vi "ClientGUIMonitorAllAnalog.vi"() -> ()   [LabVIEW 2021]
doc: "Le protocole UDP diffère du protocole TCP car il n'y a pas de détection d'erreur avec les paquets d'informations qui sont envoyés ; il n'y a donc aucune garantie qu'un destinataire reçoive bien des données.\n\nLe protocole UDP offre la possibilité de diffuser des données sur un réseau. Spécifiez simplement une adresse IP de uns (255.255.255.255) pour essayer de diffuser l'information sur tout le réseau. Gardez à l'esprit que des routeurs et d'autres périphériques de réseau refusent généralement de diffuser au-delà de certains points, la diffusion est donc limitée dans la pratique."
panel:
  out "Value":u16
  in  "?":bool
  in  "Période\n(en ds)":u32(slide)=100 min=5 max=100 step=5 scale=5.0..100.0
  out "Pin0":u16(graph)
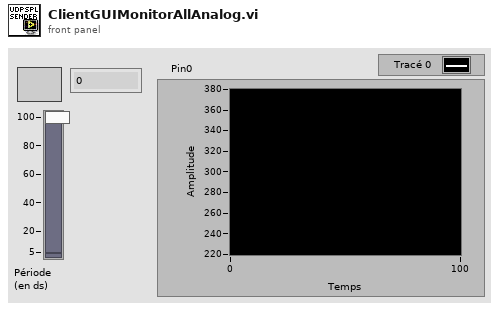
[diagram p1: front panel]
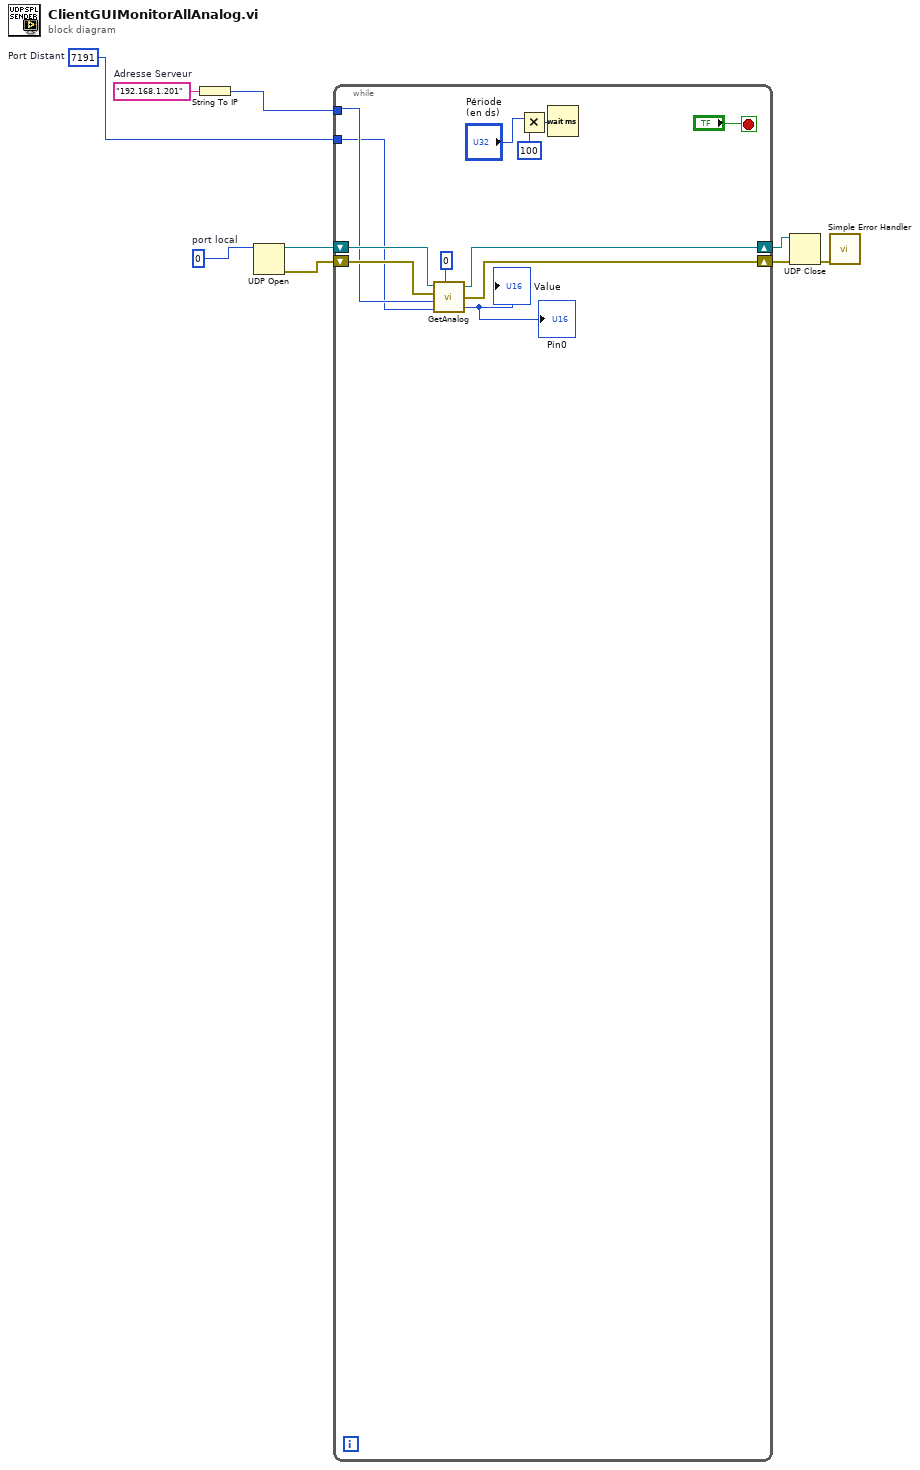
[diagram p0: block diagram]
diagram:
  w7 = u16 7191  # Port Distant
  w6 = "192.168.1.201"  # Adresse Serveur
  w9 = u16 0  # port local
  n1 = String To IP(1:w6) -> (0:w8:u32)
  n2 = UDP Open(11:w9) -> (port=w5:refnum<k16>, 0:w4:errorcluster)  [unwired: 4 in, 1 out]
  n3 = while {
    tunnel: w8 -> [w14]
    tunnel: w7 -> [w10]
    shift-right: [w13] -> w1
    shift-left: w5 -> [w16]
    shift-right: [w12] -> w2
    shift-left: w4 -> [w15]
    stop <- "?" stop-if-true
    n4 = call "GetAnalog.vi"(0:w16, 1:u8 0 ("Pin"), 2:w15, 3:w14, 5:w10) -> (6:w13:refnum<k16>, 7:w12:errorcluster, 8:→"Pin0" →"Value":u16)  [unwired: 1 in]
    n5 = Multiply(x="Période\n(en ds)", y=u32 100) -> (x*y=w19:u32)
    n6 = Wait (ms)(milliseconds to wait=w19) -> ()  [unwired: 1 out]
  }
  n7 = UDP Close(connection ID=w1, 8:w2) -> (error out=w3:errorcluster)  [unwired: 1 out]
  n8 = call <vilib>:"Simple Error Handler.vi"(9:w3) -> ()  [unwired: 4 in, 5 out]
